vi "Device Setup Testing.vi"   [LabVIEW 2013, in "Stanford Research Systems CG635.lvlib"]
uses:
  <instrlib>/Stanford Research Systems CG635/Stanford Research Systems CG635.lvlib
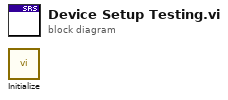
[diagram p0: block diagram]
diagram:
  n1 = call <instrlib>:"Initialize.vi"() -> ()  [unwired: 10 in, 2 out]
